vi "Stop Core.vi"(10 "final error code":i32, 11 "Power Supply in":refnum<class "Power Supply.lvclass">) -> (3 "Power Supply out":refnum<class "Power Supply.lvclass">)   [LabVIEW 2020, in "Power Supply.lvlib" / "Power Supply.lvclass"]
doc: "(<B>Filename</B>: Actor Framework.lvlib:Actor.lvclass:Stop Core.vi)\n\nDefines what the actor does before it stops. Use the <B>final error code</B> input to determine whether the actor shut down in response to an error.\n\nBy default, this method passes the Stop message along to all auto-stop nested actors. A descendant class may override this method to define additional behavior, such as shutting down any processes the actor initiated in its override of the Actor Core method."
uses:
  Power Supply.lvclass
  Power Supply.lvclass/Power Supply.ctl
  <vilib>/ActorFramework/Actor/Actor.lvclass
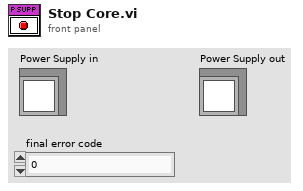
[diagram p1: front panel]
types:
  T1 = cluster{"Output Status":refnum<user-event>, "Stop":refnum<user-event>, "Status":refnum<user-event>}
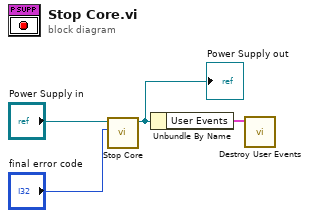
[diagram p0: block diagram]
diagram:
  n1 = call-parent "Stop Core.vi"("final error code"="final error code", "Actor in"="Power Supply in") -> ("Actor out"=w2:refnum<class "Power Supply.lvclass">)  [unwired: 9 in]
  "Power Supply out" <- w2
  n2 = Unbundle By Name(w2) -> ("User Events"=w1:T1)
  n3 = call "Destroy User Events.vi"("Cluster"=w1) -> ()  [unwired: 11 in]
